vi "RSZVB Get Calibration Kit User Connector Type With Label.vi"(8 "error in (no error)":errorcluster {"code" format="%.0x"}, 10 "Connection Type (\"\")":string, 11 "VISA session":refnum<visa-resource-name>) -> (0 "error out":errorcluster {"code" format="%.0x"}, 2 "Calibration Kit Data":string, 3 "dup VISA session":refnum<visa-resource-name>)   [LabVIEW 2011]
doc: "This VI returns the name and label of calibration kit.\n\nRemote-control command(s):\n[SENSe<Ch>:]CORRection:CKIT:LSELect? '<conn_type>'"
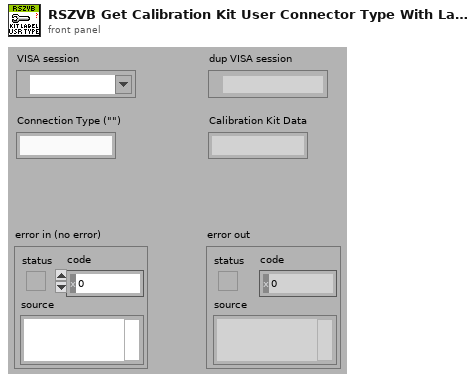
[diagram p1: front panel]
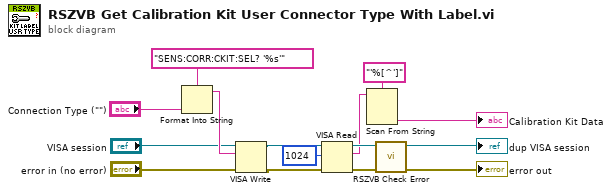
[diagram p0: block diagram]
diagram:
  n1 = Format Into String(format string="SENS:CORR:CKIT:SEL? '%s'", "Connection Type (\"\")") -> (resulting string=w14:string)  [unwired: 2 in, 1 out]
  n2 = VISA Write(VISA resource name="VISA session", write buffer=w14, error in (no error)="error in (no error)") -> (VISA resource name out=w9:refnum<visa-resource-name>, error out=w8:errorcluster)  [unwired: 1 out]
  n3 = VISA Read(VISA resource name=w9, byte count=u32 1024 ("byte count (0)"), error in (no error)=w8) -> (VISA resource name out=w13:refnum<visa-resource-name>, read buffer=w10:string, error out=w12:errorcluster)  [unwired: 1 out]
  n4 = Scan From String(format string="'%[^']", input string=w10) -> (output 1=→"Calibration Kit Data":string)  [unwired: 3 in, 3 out]
  n5 = call "RSZVB Check Error.vi"("error in (no error)"=w12, "VISA session"=w13) -> ("error out"=→"error out":errorcluster, "dup VISA session"=→"dup VISA session":refnum<visa-resource-name>)  [unwired: 8 in]
